vi "run.vi"(8 "error in (no error)":errorcluster, 11 "DL090624AnalyserScaffold in":refnum<class "AnalyserDL090624Scaffold.lvclass">) -> (0 "error out":errorcluster, 3 "DL090624AnalyserScaffold out":refnum<class "AnalyserDL090624Scaffold.lvclass">)   [LabVIEW 2010, in "AnalyserDL090624Scaffold.lvclass"]
uses:
  AnalyserDL090624Scaffold.lvclass
  GenericAnalyser/GenericAnalyser/GenericAnalyser.lvclass
  common/classes/ErrorController/ErrorController/class_data.vi
  common/classes/ErrorController/ErrorController/ErrorController.lvclass
panel:
  out "statechart loop counter":i32
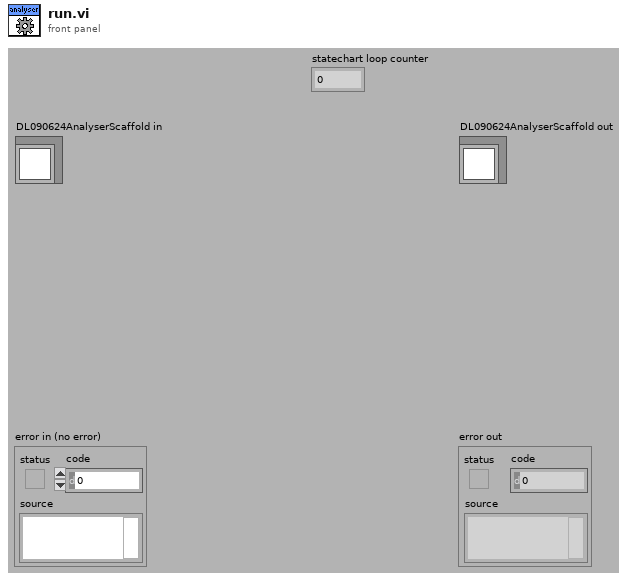
[diagram p1: front panel]
types:
  T1 = typedef "GenericToplevelComponent.lvclass/common_trigger_enum.ctl" = enum16{"NULL", "initialise", "terminate", "fetch command", "fetch data", "attach observer", "register as observer", "detach observer", "acknowledge", "start", "stop", "sweep started", "sweep finished", "experiment started", "experiment stopped"}
  T2 = typedef "AnalyserDL090624Scaffold.lvclass/internal_trigger_enum.ctl" = enum16{"NULL", "initialise", "terminate", "start", "stop", "analyse", "register as observer"}
  T3 = typedef "main_trigger_enum.ctl" = enum16{"NULL", "initialise", "terminate", "start", "stop", "change objective", "change experimentController", "change imagingMode", "save notebook", "started saving", "finished saving", "expCtr ready", "expCtr missing", "imgMd ready", "imgMd missing", "scanHd ready", "scanHd missing", "DAQ ready", "DAQ missing", "imgAsm ready", "imgAsm missing", "dataColl ready", "dataColl missing", "display ready", "display missing", "analysr ready", "analysr missing", "instrmnt ready", "instrmnt missing", "stimltr ready", "stimltr missing", "stage ready", "stage missing"}
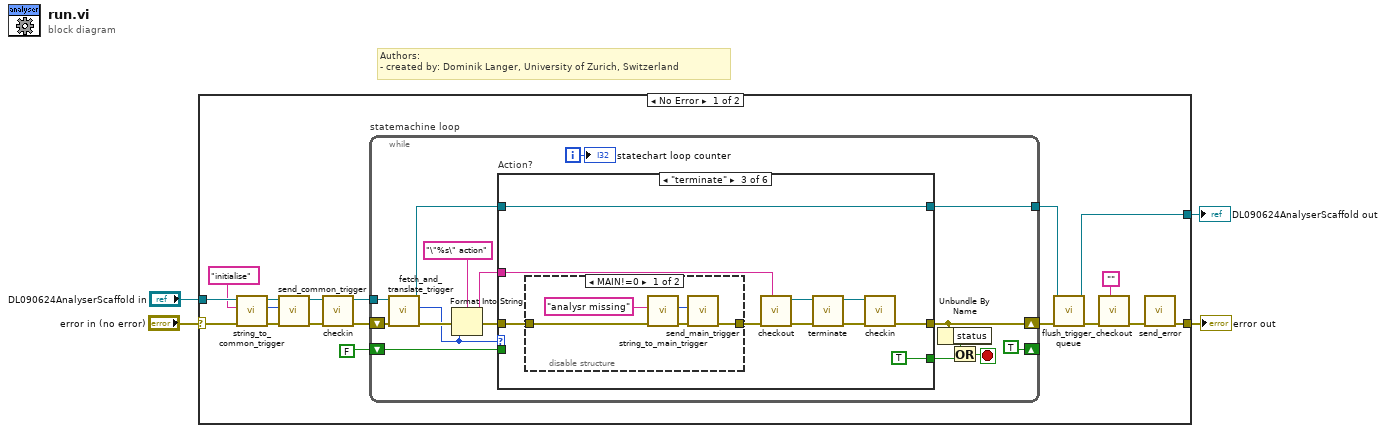
[diagram p0: block diagram]
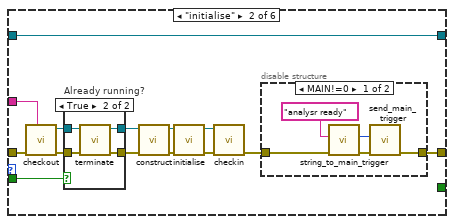
[diagram p3: hidden frame]
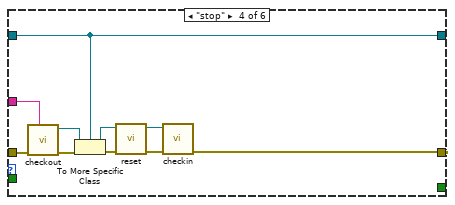
[diagram p7: hidden frame]
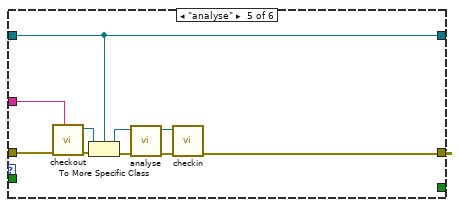
[diagram p8: hidden frame]
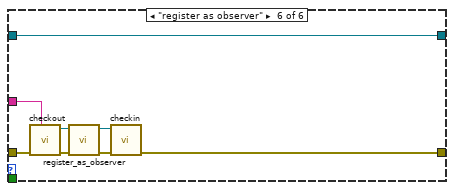
[diagram p9: hidden frame]
diagram:
  # "Authors: \n- created by: Dominik Langer, University of Zurich, Switzerland"
  n1 = case shown="No Error" "error in (no error)" {
    selector: "error in (no error)" -> [w10 w112]
    tunnel: [w18 w112] -> w3
    tunnel: [w13 w111] -> w1
    tunnel: "DL090624AnalyserScaffold in" -> [w8 w111]
    frame No Error {
      n2 = call-dynamic "string_to_common_trigger.vi"("error in (no error)"=w10, "trigger string"="initialise", "GenericToplevelComponent in"=w8) -> ("error out"=w9:errorcluster, "trigger"=w6:T1, "GenericToplevelComponent out"=w7:refnum<class "AnalyserDL090624Scaffold.lvclass">)  [unwired: 6 in]
      n3 = call-dynamic "send_common_trigger.vi"("error in (no error)"=w9, "trigger"=w6, "GenericToplevelComponent in"=w7) -> ("error out"=w12:errorcluster, "GenericToplevelComponent out"=w11:refnum<class "AnalyserDL090624Scaffold.lvclass">)  [unwired: 6 in, 1 out]
      n4 = call-dynamic "checkin.vi"("error in (no error)"=w12, "GeneralAnalyser in"=w11) -> ("error out"=w22:errorcluster, "GeneralAnalyser out"=w17:refnum<class "AnalyserDL090624Scaffold.lvclass">)  [unwired: 8 in]
      n5 = while "statemachine loop" {
        shift-right: [TRUE] -> _
        shift-left: FALSE -> [w27]
        tunnel: w17 -> [w34]
        shift-right: [w24] -> w16
        shift-left: w22 -> [w35]
        tunnel: [w25] -> w14
        i -> [w38]
        stop <- w36 stop-if-true
        n6 = call-dynamic "fetch_and_translate_trigger.vi"("error in (no error)"=w35, "AnalyserDL090624Scaffold in"=w34) -> ("error out"=w32:errorcluster, "trigger"=w30:T2, "AnalyserDL090624Scaffold out"=w33:refnum<class "AnalyserDL090624Scaffold.lvclass">)  [unwired: 6 in, 1 out]
        n7 = Format Into String(format string="\"%s\" action", error in=w32, w30) -> (resulting string=w28:string, error out=w31:errorcluster)  [unwired: 1 in]
        n8 = case "Action?" shown="\"terminate\"" w30 {
          tunnel: w31 -> [w40 w52 w70 w88 w96 w105]
          tunnel: [w40 w42 w72 w83 w93 w104] -> w24
          tunnel: w33 -> [w39 w41 w67 w86 w95 w103]
          tunnel: w28 -> [_ w49 w71 w89 w94 w106]
          tunnel: w27 -> [_ w44 _ _ _ _]
          tunnel: [_ _ TRUE _ _ _] -> w26
          tunnel: [w39 w41 w67 w86 w95 w103] -> w25
          frame "NULL", Default {
          }
          frame "initialise" {
            n9 = call "checkout.vi"("locked by?"=w49, "error in (no error)"=w52) -> ("error out"=w48:errorcluster, "GeneralAnalyser out"=w46:refnum<class "GenericAnalyser.lvclass">)  [unwired: 8 in]
            n10 = case "Already running?" shown="True" w44 {
              tunnel: w48 -> [w61 w66]
              tunnel: [w61 w65] -> w47
              tunnel: w46 -> [w62 w64]
              tunnel: [w62 w63] -> w45
              frame False {
              }
              frame True {
                n11 = call-dynamic "terminate.vi"("error in (no error)"=w66, "GenericPlugin in"=w64) -> ("error out"=w65:errorcluster, "GenericPlugin out"=w63:refnum<class "GenericAnalyser.lvclass">)  [unwired: 8 out]
              }
            }
            n12 = call-dynamic "construct.vi"("error in (no error)"=w47, "GenericPlugin in"=w45) -> ("error out"=w50:errorcluster, "GenericPlugin out"=w54:refnum<class "GenericAnalyser.lvclass">)  [unwired: 2 in, 6 out]
            n13 = call-dynamic "initialise.vi"("error in (no error)"=w50, "GenericPlugin in"=w54) -> ("error out"=w51:errorcluster, "GenericPlugin out"=w53:refnum<class "GenericAnalyser.lvclass">)  [unwired: 8 out]
            n14 = call-dynamic "checkin.vi"("error in (no error)"=w51, "GeneralAnalyser in"=w53) -> ("error out"=w43:errorcluster)  [unwired: 8 in, 1 out]
            n15 = disable-structure shown="MAIN!=0" {
              disable-tunnel: w43 -> [w58 w60]
              disable-tunnel: [w59 w60] -> w42
              frame condition #0 (active) {
                n16 = call "string_to_main_trigger.vi"("error in (no error)"=w58, "trigger string"="analysr ready" ("input string")) -> ("error out"=w57:errorcluster, "main trigger"=w56:T3)  [unwired: 8 in]
                n17 = call "send_main_trigger.vi"("error in (no error)"=w57, "trigger"=w56) -> ("error out"=w59:errorcluster)  [unwired: 9 in]
              }
              frame condition #1 {
              }
            }
          }
          frame "terminate" {
            n18 = disable-structure shown="MAIN!=0" {
              disable-tunnel: w70 -> [w79 w82]
              disable-tunnel: [w77 w82] -> w69
              frame condition #0 (active) {
                n19 = call "string_to_main_trigger.vi"("error in (no error)"=w79, "trigger string"="analysr missing" ("input string")) -> ("error out"=w80:errorcluster, "main trigger"=w81:T3)  [unwired: 8 in]
                n20 = call "send_main_trigger.vi"("error in (no error)"=w80, "trigger"=w81) -> ("error out"=w77:errorcluster)  [unwired: 9 in]
              }
              frame condition #1 {
              }
            }
            n21 = call "checkout.vi"("locked by?"=w71, "error in (no error)"=w69) -> ("error out"=w74:errorcluster, "GeneralAnalyser out"=w76:refnum<class "GenericAnalyser.lvclass">)  [unwired: 8 in]
            n22 = call-dynamic "terminate.vi"("error in (no error)"=w74, "GenericPlugin in"=w76) -> ("error out"=w73:errorcluster, "GenericPlugin out"=w75:refnum<class "GenericAnalyser.lvclass">)  [unwired: 8 out]
            n23 = call-dynamic "checkin.vi"("error in (no error)"=w73, "GeneralAnalyser in"=w75) -> ("error out"=w72:errorcluster)  [unwired: 8 in, 1 out]
          }
          frame "stop" {
            n24 = call "checkout.vi"("locked by?"=w89, "error in (no error)"=w88) -> ("error out"=w87:errorcluster, "GeneralAnalyser out"=w92:refnum<class "GenericAnalyser.lvclass">)  [unwired: 8 in]
            n25 = To More Specific Class(target class=w86, reference=w92, error in=w87) -> (specific class reference=w90:refnum<class "AnalyserDL090624Scaffold.lvclass">, error out=w85:errorcluster)
            n26 = call-dynamic "reset.vi"("error in (no error)"=w85, "DL090624AnalyserScaffold in"=w90) -> ("error out"=w84:errorcluster, "DL090624AnalyserScaffold out"=w91:refnum<class "AnalyserDL090624Scaffold.lvclass">)  [unwired: 8 out]
            n27 = call-dynamic "checkin.vi"("error in (no error)"=w84, "GeneralAnalyser in"=w91) -> ("error out"=w83:errorcluster)  [unwired: 8 in, 1 out]
          }
          frame "analyse" {
            n28 = call "checkout.vi"("locked by?"=w94, "error in (no error)"=w96) -> ("error out"=w102:errorcluster, "GeneralAnalyser out"=w101:refnum<class "GenericAnalyser.lvclass">)  [unwired: 8 in]
            n29 = To More Specific Class(target class=w95, reference=w101, error in=w102) -> (specific class reference=w99:refnum<class "AnalyserDL090624Scaffold.lvclass">, error out=w100:errorcluster)
            n30 = call-dynamic "analyse.vi"("error in (no error)"=w100, "DL090624AnalyserScaffold in"=w99) -> ("error out"=w98:errorcluster, "DL090624AnalyserScaffold out"=w97:refnum<class "AnalyserDL090624Scaffold.lvclass">)  [unwired: 8 out]
            n31 = call-dynamic "checkin.vi"("error in (no error)"=w98, "GeneralAnalyser in"=w97) -> ("error out"=w93:errorcluster)  [unwired: 8 in, 1 out]
          }
          frame "register as observer" {
            n32 = call "checkout.vi"("locked by?"=w106, "error in (no error)"=w105) -> ("error out"=w110:errorcluster, "GeneralAnalyser out"=w108:refnum<class "GenericAnalyser.lvclass">)  [unwired: 8 in]
            n33 = call-dynamic "register_as_observer.vi"("error in (no error)"=w110, "GenericToplevelComponent in"=w108) -> ("error out"=w109:errorcluster, "GenericToplevelComponent out"=w107:refnum<class "GenericAnalyser.lvclass">)  [unwired: 8 in]
            n34 = call-dynamic "checkin.vi"("error in (no error)"=w109, "GeneralAnalyser in"=w107) -> ("error out"=w104:errorcluster)  [unwired: 8 in, 1 out]
          }
        }
        n35 = Unbundle By Name(w24) -> ("status"=w23:bool)
        n36 = Or(x=w23, y=w26) -> (x .or. y?=w36:bool)
        "statechart loop counter" <- w38
      }
      n37 = call-dynamic "flush_trigger_queue.vi"("error in (no error)"=w16, "GenericToplevelComponent in"=w14) -> ("error out"=w15:errorcluster, "GenericToplevelComponent out"=w13:refnum<class "AnalyserDL090624Scaffold.lvclass">)  [unwired: 8 in]
      n38 = call "checkout.vi"("locked by?"="", "error in (no error)"=w15) -> ("error out"=w19:errorcluster)  [unwired: 8 in, 1 out]
      n39 = call "send_error.vi"("error in (no error)"=w19) -> ("error out"=w18:errorcluster)  [unwired: 10 in]
    }
    frame Error {
    }
  }
  "error out" <- w3
  "DL090624AnalyserScaffold out" <- w1
